vi "getMessage.vi"(8 "error in (no error)":errorcluster, 11 "TCPClient in":refnum<class "TCPClient.lvclass">) -> (0 "error out":errorcluster, 2 "String":string, 3 "TCPClient out":refnum<class "TCPClient.lvclass">)   [LabVIEW 2016, in "TCPClient.lvclass"]
uses:
  TCPClient.lvclass
  TCPSettings/TCPSettings.lvclass
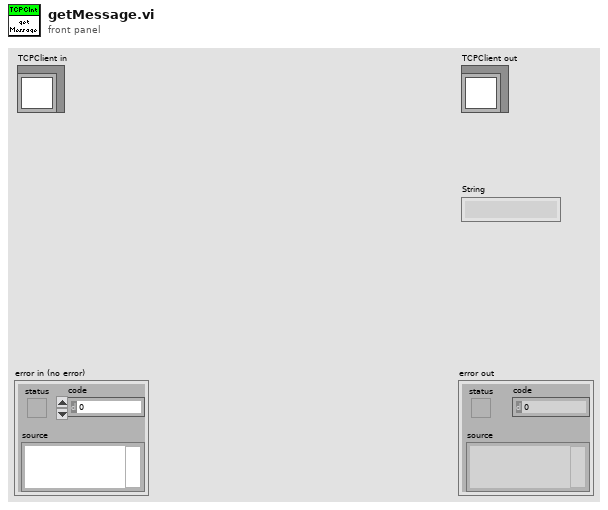
[diagram p1: front panel]
types:
  T1 = enum16{"Standard", "Buffered", "CRLF", "Immediate"}
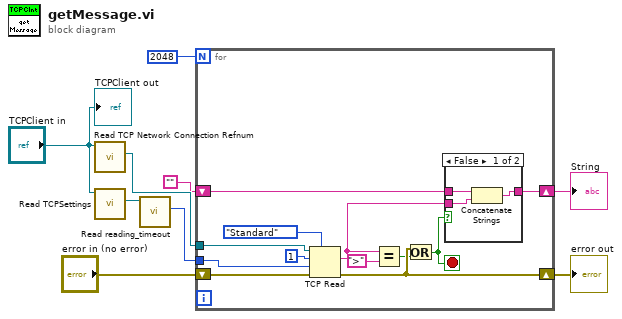
[diagram p0: block diagram]
diagram:
  n1 = call-dynamic "Read TCP Network Connection Refnum.vi"("TCPCommunicator in"="TCPClient in") -> ("TCP Network Connection Refnum"=w8:refnum<k5>)  [unwired: 8 in, 2 out]
  n2 = call-dynamic "Read TCPSettings.vi"("TCPCommunicator in"="TCPClient in") -> ("TCPSettings.lvclass"=w7:refnum<class "TCPSettings.lvclass">)  [unwired: 8 in, 2 out]
  n3 = call-dynamic "Read reading_timeout.vi"("TCPSettings in"=w7) -> ("reading_timeout"=w9:i32)  [unwired: 8 in, 2 out]
  n4 = for {
    N: 2048 -> [_]
    tunnel: w9 -> [w21]
    tunnel: w8 -> [w20]
    shift-right: [w16] -> w3
    shift-left: "error in (no error)" -> [w19]
    shift-right: [w14] -> w6
    shift-left: "" ("String") -> [w15]
    stop <- w10 stop-if-true
    n5 = TCP Read(connection ID=w20, bytes to read=1, error in (no error)=w19, 7:T1."Standard" ("mode (standard)"), 9:w21) -> (data out=w13:string, error out=w16:errorcluster)  [unwired: 1 out]
    n6 = Equal?(x=w13, y=">") -> (x = y?=w11:bool)
    n7 = Or(x=w16, y=w11) -> (x .or. y?=w10:bool)
    n8 = case shown="False" w10 {
      tunnel: w15 -> [w24 w25]
      tunnel: [w23 w25] -> w14
      tunnel: w13 -> [w22 _]
      frame False {
        n9 = Concatenate Strings(w24, w22) -> (w23:string)
      }
      frame True {
      }
    }
  }
  "error out" <- w3
  "String" <- w6
  "TCPClient out" <- "TCPClient in"
